vi "density.vi"(8 "error in (no error)":errorcluster, 10 "pPa":dbl, 11 "TK":dbl) -> (0 "error out":errorcluster, 3 "function return":dbl)   [LabVIEW 2011, in "fsteam.lvlib"]
doc: "extern double density(double TK, double pPa);"
uses:
  <userlib>/fsteam/fsteam.lvlib
  <userlib>/fsteam/fsteam.dll
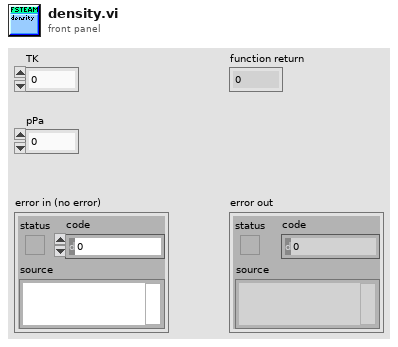
[diagram p1: front panel]
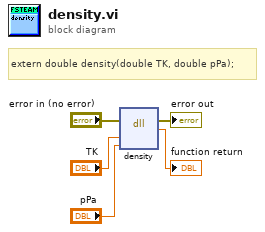
[diagram p0: block diagram]
diagram:
  # "extern double density(double TK, double pPa);"
  n1 = dll-call lib="C:/Program Files (x86)/National Instruments/LabVIEW 2011/user.lib/fsteam/fsteam.*" fn="density"(error in="error in (no error)", "TK"="TK", "pPa"="pPa") -> (error out=→"error out":errorcluster, →"function return":dbl)  [unwired: 4 in, 1 out]
